vi "Monitors_v02.vi"(8 "wfm":waveform(dbl)[](array[waveform]), 9 "Shot noise start":bool, 10 "Monitor Switches":T1, 11 "IIR filter specifications":T2={"Topology"=enum."Butterworth", "Type"=enum."Lowpass", "Order"=1, "Lower Fc"=100.0, "Upper Fc"=200.0, "PB Ripple"=1.0, "SB Attenuation"=60.0} {"PB Ripple" format="%0.2f"; "SB Attenuation" format="%0.2f"; "Lower Fc" format="%0.2p"; "Upper Fc" format="%0.2p"}) -> (0 "covariance":dbl, 1 "conditional variance":dbl, 2 "Variance 2 normalised to SNL":dbl(graph), 3 "Variance 1 normalised to SNL":dbl(graph))   [LabVIEW 2013]
uses:
  Strict Type Defs/Monitor switches.ctl
  <vilib>/Analysis/5stat.llb/RMS (DBL).vi
  <vilib>/Analysis/baseanly.llb/Mean (DBL).vi
  <vilib>/measure/macond.llb/IIR Filter for N Chan.vi
  Global VIs/shotnoise.vi
  <vilib>/measure/NI_MAPro.lvlib
  <vilib>/Analysis/NI_AALPro.lvlib
  <vilib>/Analysis/NI_AALBase.lvlib
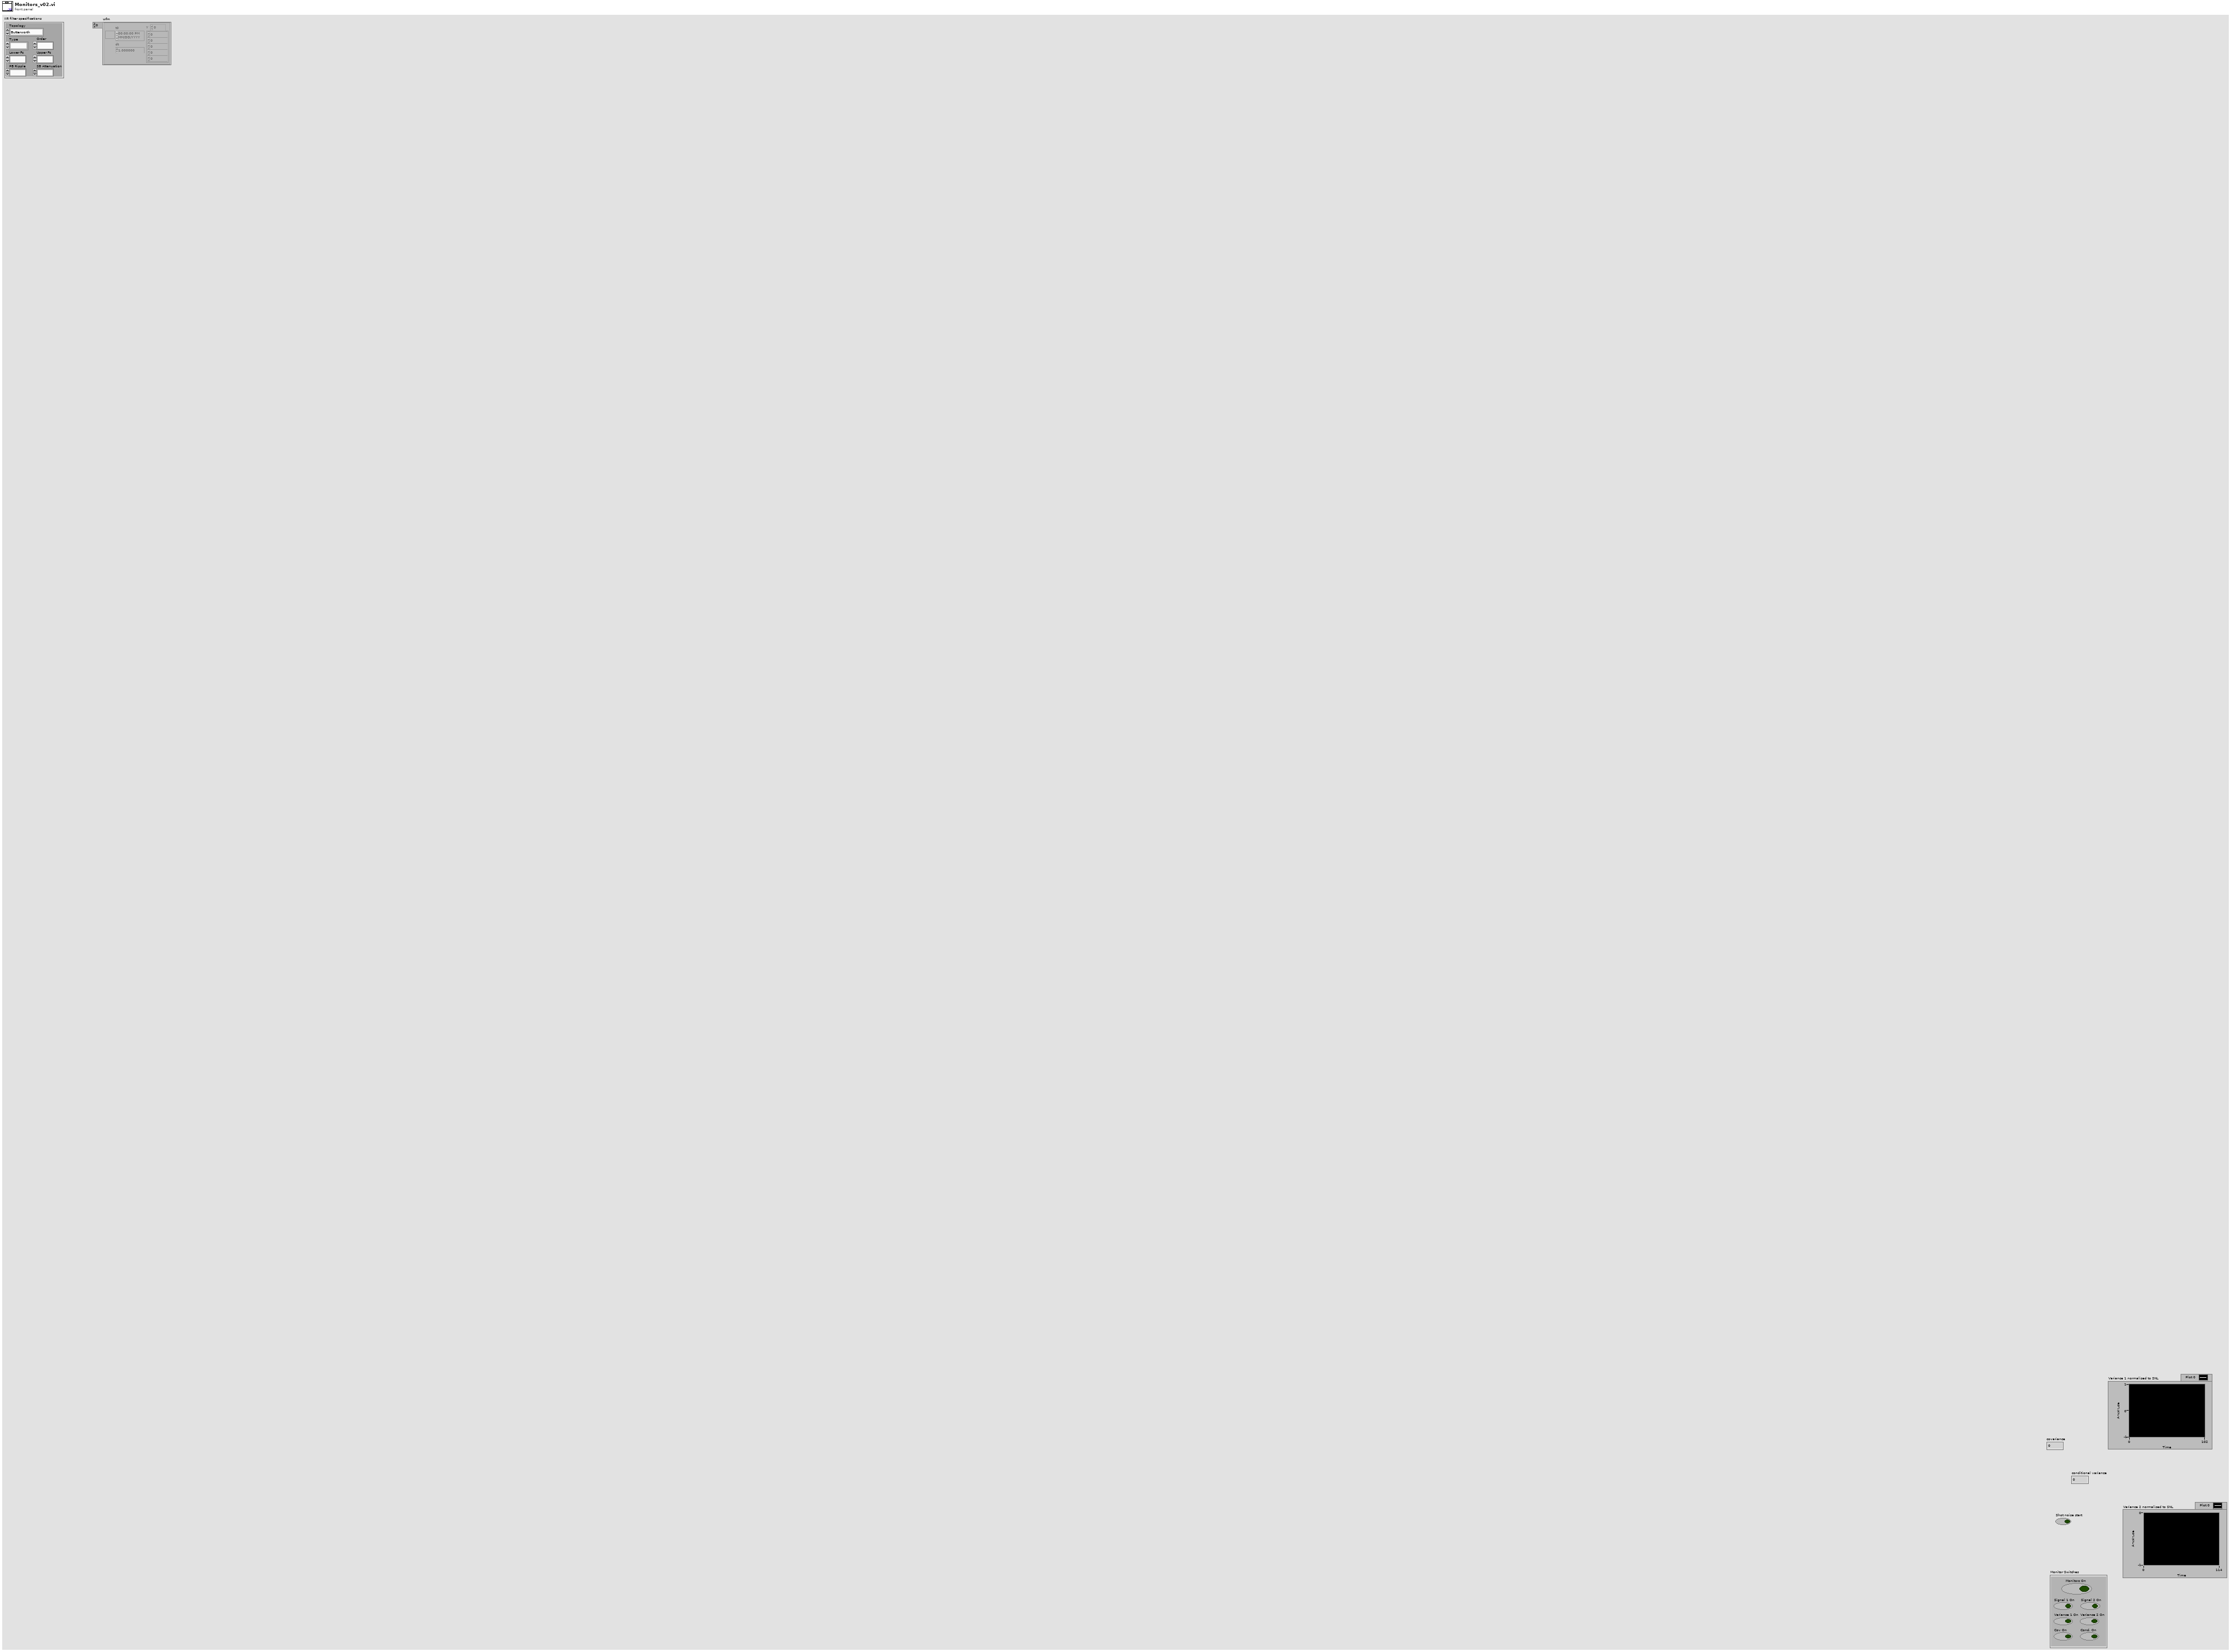
[diagram p1: front panel]
types:
  T1 = typedef "Monitor switches.ctl" = cluster{"Signal 1 On":bool, "Signal 2 On":bool, "Variance 1 On":bool, "Variance 2 On":bool, "Cov On":bool, "Cond. On":bool, "Monitors On":bool}
  T2 = cluster{"Topology":enum16{"Off", "Butterworth", "Chebyshev", "Inverse Chebyshev", "Elliptic", "Bessel"}, "Type":enum16{"Lowpass", "Highpass", "Bandpass", "Bandstop"}, "Order":i32, "Lower Fc":dbl, "Upper Fc":dbl, "PB Ripple":dbl, "SB Attenuation":dbl}
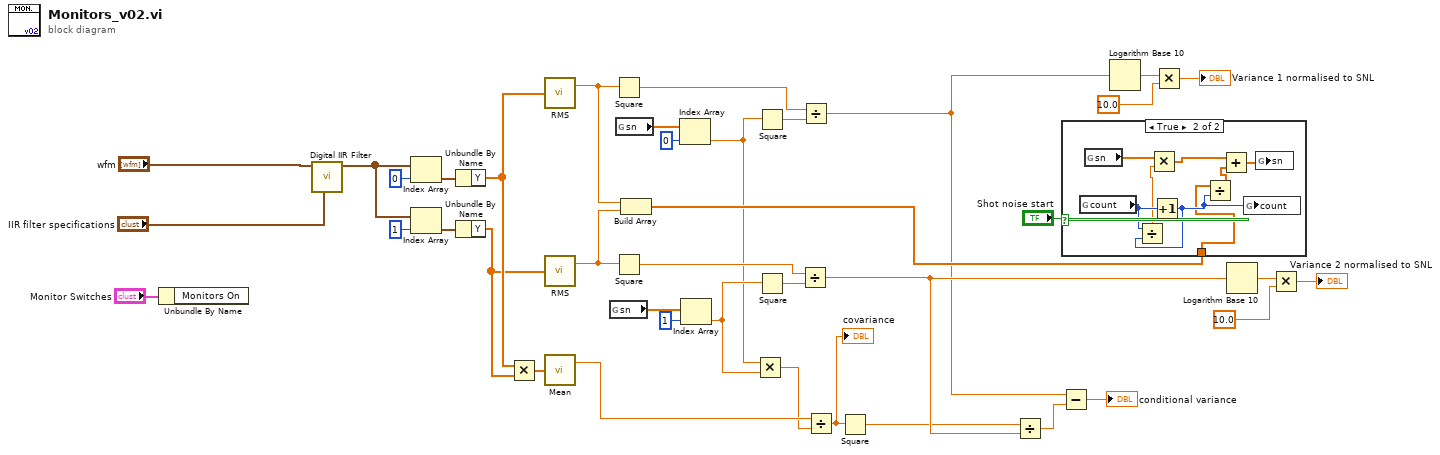
[diagram p0: block diagram]
diagram:
  n1 = Unbundle By Name("Monitor Switches") -> ()  [unwired: 1 out]
  n2 = call-poly <vilib>:"Digital IIR Filter.vi"("IIR filter specifications"="IIR filter specifications", "signal(s) in"="wfm") -> ("signal(s) out"=w1:waveform(dbl)[])  [unwired: 4 in, 5 out]
  n3 = Index Array(array=w1, index=0) -> (element=w10:waveform(dbl))
  n4 = Index Array(array=w1, index=1) -> (element=w15:waveform(dbl))
  n5 = Unbundle By Name(w10) -> ("Y"=w35:dbl[])
  n6 = Unbundle By Name(w15) -> ("Y"=w30:dbl[])
  n7 = Multiply(x=w35, y=w30) -> (x*y=w33:dbl[])
  n8 = call-poly <vilib>:"RMS.vi"("X"=w35) -> ("rms value"=w28:dbl)  [unwired: 1 out]
  n9 = call-poly <vilib>:"RMS.vi"("X"=w30) -> ("rms value"=w31:dbl)  [unwired: 1 out]
  n10 = call-poly <vilib>:"Mean.vi"("X"=w33) -> ("mean"=w34:dbl)  [unwired: 1 out]
  n11 = global read "shotnoise.vi" "sn"() -> (w13:dbl[])
  n12 = Square(x=w28) -> (x^2=w29:dbl)
  n13 = Square(x=w31) -> (x^2=w32:dbl)
  n14 = global read "shotnoise.vi" "sn"() -> (w12:dbl[])
  n15 = Build Array(w28, w31) -> (w27:dbl[])
  n16 = Index Array(array=w12, index=0) -> (element=w23:dbl)
  n17 = Index Array(array=w13, index=1) -> (element=w24:dbl)
  n18 = Multiply(x=w23, y=w24) -> (x*y=w25:dbl)
  n19 = Square(x=w23) -> (x^2=w20:dbl)
  n20 = Square(x=w24) -> (x^2=w22:dbl)
  n21 = Divide(x=w32, y=w22) -> (x/y=w26:dbl)
  n22 = Divide(x=w29, y=w20) -> (x/y=w21:dbl)
  n23 = Divide(x=w34, y=w25) -> (x/y=w36:dbl)
  "covariance" <- w36
  n24 = Square(x=w36) -> (x^2=w17:dbl)
  n25 = Divide(x=w17, y=w26) -> (x/y=w18:dbl)
  n26 = Subtract(x=w21, y=w18) -> (x-y=→"conditional variance":dbl)
  n27 = case shown="True" "Shot noise start" {
    tunnel: w27 -> [_ w41]
    frame False {
    }
    frame True {
      n28 = global read "shotnoise.vi" "count"() -> (w46:i64)
      n29 = global read "shotnoise.vi" "sn"() -> (w45:dbl[])
      n30 = Increment(x=w46) -> (x+1=w42:i64)
      n31 = Divide(x=w46, y=w42) -> (x/y=w44:dbl)
      n32 = Multiply(x=w45, y=w44) -> (x*y=w43:dbl[])
      n33 = Divide(x=w41, y=w42) -> (x/y=w40:dbl[])
      n34 = Add(x=w43, y=w40) -> (x+y=w47:dbl[])
      n35 = global write "shotnoise.vi" "count"(w42) -> ()
      n36 = global write "shotnoise.vi" "sn"(w47) -> ()
    }
  }
  n37 = Logarithm Base 10(1:w21) -> (0:w2:dbl)
  n38 = Multiply(x=w2, y=10.0) -> (x*y=→"Variance 1 normalised to SNL":dbl)
  n39 = Logarithm Base 10(1:w26) -> (0:w5:dbl)
  n40 = Multiply(x=w5, y=10.0) -> (x*y=→"Variance 2 normalised to SNL":dbl)
